vi "Create.vi"(8 "error in (no error)":errorcluster, 11 "GPS in":refnum<class "GPS.lvclass">) -> (0 "error out":errorcluster, 3 "GPS out":refnum<class "GPS.lvclass">)   [LabVIEW 2020, in "GPS.lvlib" / "GPS.lvclass"]
uses:
  GPS.lvclass
  C:/Users/dzoni/Documents/NJ/Playground/LV/TCP GPS/src/ClientBase/TCP.lvclass
  TCP/TCP.lvclass
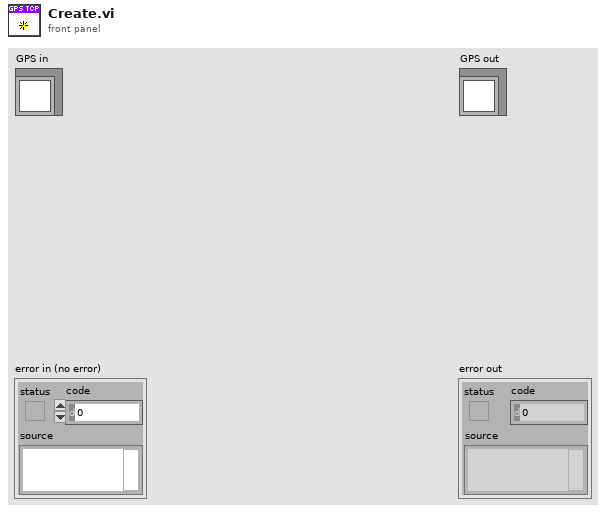
[diagram p1: front panel]
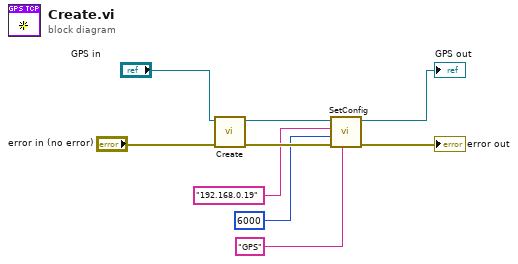
[diagram p0: block diagram]
diagram:
  n1 = call-parent "Create.vi"("error in (no error)"="error in (no error)", "ClientBase in"="GPS in") -> ("error out"=w5:errorcluster, "ClientBase out"=w7:refnum<class "GPS.lvclass">)  [unwired: 8 in]
  n2 = call "SetConfig.vi"("ID"="GPS", "error in (no error)"=w5, "Port"=u16 6000, "Address"="192.168.0.19", "ClientBase in"=w7) -> ("error out"=→"error out":errorcluster, "ClientBase out"=→"GPS out":refnum<class "GPS.lvclass">)  [unwired: 5 in]
